vi "OutputRF.vi"(6 "Route Names":string[](array[string]), 7 "output enabled":bool=TRUE, 8 "error in (no error)":errorcluster, 9 "Power (dBm)":dbl, 10 "Frequency (Hz)":dbl, 11 "SigGen_ESG in":refnum<class "SigGen_ESG.lvclass">) -> (0 "error out":errorcluster, 3 "SigGen_ESG out":refnum<class "SigGen_ESG.lvclass">)   [LabVIEW 2014, in "SigGen_ESG.lvclass"]
uses:
  SigGen_ESG.lvclass
  SigGen_ESG.lvclass/SigGen_ESG.ctl
  <instrlib>/Agilent ESG Series/Agilent ESG Series.lvlib
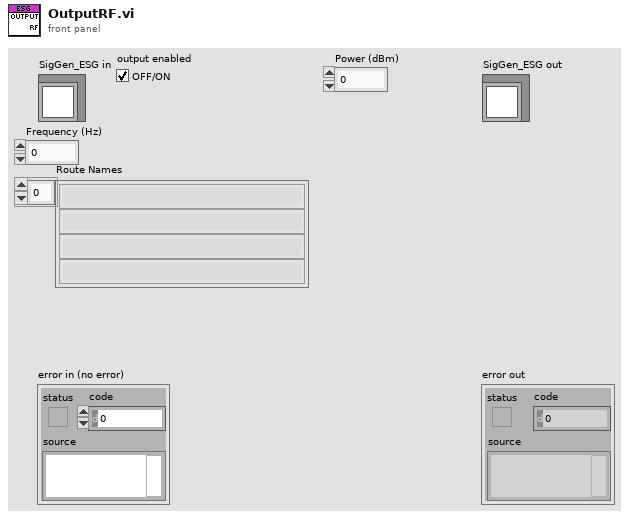
[diagram p1: front panel]
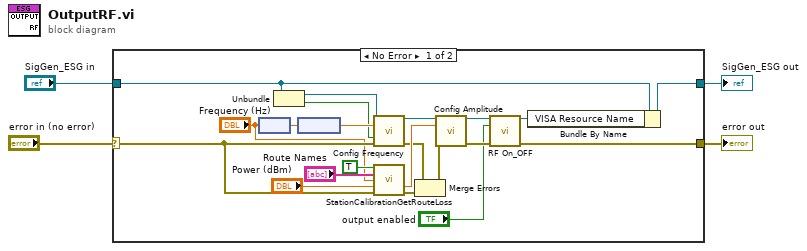
[diagram p0: block diagram]
diagram:
  n1 = case shown="No Error" "error in (no error)" {
    selector: "error in (no error)" -> [w19 w27]
    tunnel: "SigGen_ESG in" -> [w10 w26]
    tunnel: [w8 w27] -> w2
    tunnel: [w7 w26] -> w1
    frame No Error {
      n2 = node("Frequency (Hz)") -> (w25:dbl[unit])
      n3 = Unbundle(w10) -> (w14:refnum<visa-resource-name>, w12:bool)
      n4 = node(w25) -> (w20:dbl)
      n5 = call <instrlib>:"Config Frequency.vi"("VISA Resource Name"=w14, "Frequency (1000.0)"=w20, "Freq Ref (T:ON)"=w12, "error in (no error)"=w19) -> ("VISA Resource Name Out"=w15:refnum<visa-resource-name>, "error out"=w17:errorcluster)  [unwired: 10 in]
      n6 = call "StationCalibrationGetRouteLoss.vi"("Calibration Enabled"=TRUE, "Route Names"="Route Names", "Frequency"="Frequency (Hz)", "Power Level"="Power (dBm)", "error in (no error)"=w19) -> ("Adjusted Power Level"=w21:dbl, "error out"=w18:errorcluster)  [unwired: 7 in, 2 out]
      n7 = Merge Errors(w17, w18) -> (w16:errorcluster)
      n8 = call <instrlib>:"Config Amplitude.vi"("VISA Resource Name"=w15, "Amplitude (-135.00)"=w21, "error in (no error)"=w16) -> ("VISA Resource Name Out"=w13:refnum<visa-resource-name>, "error out"=w11:errorcluster)  [unwired: 11 in]
      n9 = call <instrlib>:"RF On_OFF.vi"("VISA Resource Name"=w13, "Status (T:ON)"="output enabled", "error in (no error)"=w11) -> ("VISA Resource Name Out"=w9:refnum<visa-resource-name>, "error out"=w8:errorcluster)  [unwired: 11 in]
      n10 = Bundle By Name(cluster=w10, "VISA Resource Name"=w9) -> (w7:refnum<class "SigGen_ESG.lvclass">)
    }
    frame Error {
    }
  }
  "error out" <- w2
  "SigGen_ESG out" <- w1
